vi "checkBeginPassToStrikerPlay.vi"(8 "error in (no error)":errorcluster, 10 "Game":refnum<class "Game.lvclass">, 11 "PassToStriker in":refnum<class "PassToStriker.lvclass">) -> (0 "error out":errorcluster, 2 "result":bool, 3 "PassToStriker out":refnum<class "PassToStriker.lvclass">)   [LabVIEW 2018, in "PassToStrikerPlay.lvclass"]
uses:
  PassToStrikerPlay.lvclass
  temp test/PassToStriker_class/PassToStriker.lvclass
  Game_class/Game.lvclass
  Utilities_class/Utilities.lvclass
  Game_class/Game.lvclass/Game.ctl
  Team_class/Team.lvclass/Team.ctl
  Referee_class/Referee.lvclass/Referee.ctl
  Referee_class/command_interpreted.ctl
  Team_class/OffensivePlay.ctl
  Game_class/Read AllyRef.vi
  Team_class/Read RobotRef.vi
  Game_class/Read Referee.vi
  Referee_class/Read command_interpreted.vi
  Game_class/Read OffensiveTeam.vi
  Team_class/Read OffensivePlay.vi
  Ally_class/Ally.lvclass
  C:/Users/anton/Desktop/roboime/Babulho do Testoni/SSL_AI/Team_class/Team.lvclass
  Referee_class/Referee.lvclass
  Robot_class/Robot.lvclass
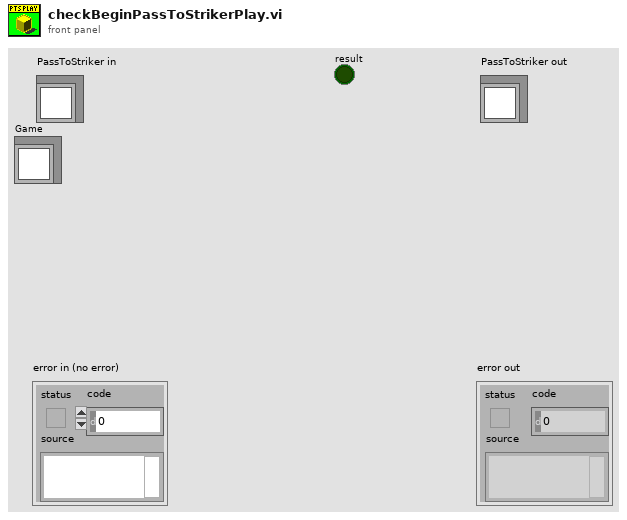
[diagram p1: front panel]
types:
  T1 = typedef "OffensivePlay.ctl" = enum16{"PreparePass", "PassToStriker", "BallOutOfField", "PassTo2ndStriker", "StopOffensive", "Prepare Penalty Enemy", "EnemyPossessionAtEnemyField", "EnemyPossesionAtOurField", "TestPlay", "PreparePenaltyAlly", "KickPenaltyAlly", "PrepareKickoffAlly", "PrepareKickoffEnemy", "IndirectEnemy", "DirectEnemy", "NormalGame", "DirectKick", "Pass", "Halt", "Timeout", "PassPlay", "PenaltyEnemy"}
  T2 = typedef "command_interpreted.ctl" = enum16{"Goal Ally", "Goal Enemy", "Ball Placement Enemy", "Ball Placement Ally", "Normal Half Time", "Extra Time  Break", "Extra Half Time", "None", "Post Game", "PKA Normal Start", "Prepare Kickoff Ally", "PKE Normal Start", "Prepare Kickoff Enemy", "Force Start", "Halt", "Timeout", "Prepare Penalty Ally", "Prepare Penalty Enemy", "PPA NormalStart", "PPE Normal Start", "Indirect Free Ally", "Direct Free Enemy", "Direct Free Ally", "Indirect Free Enemy", "Stop"}
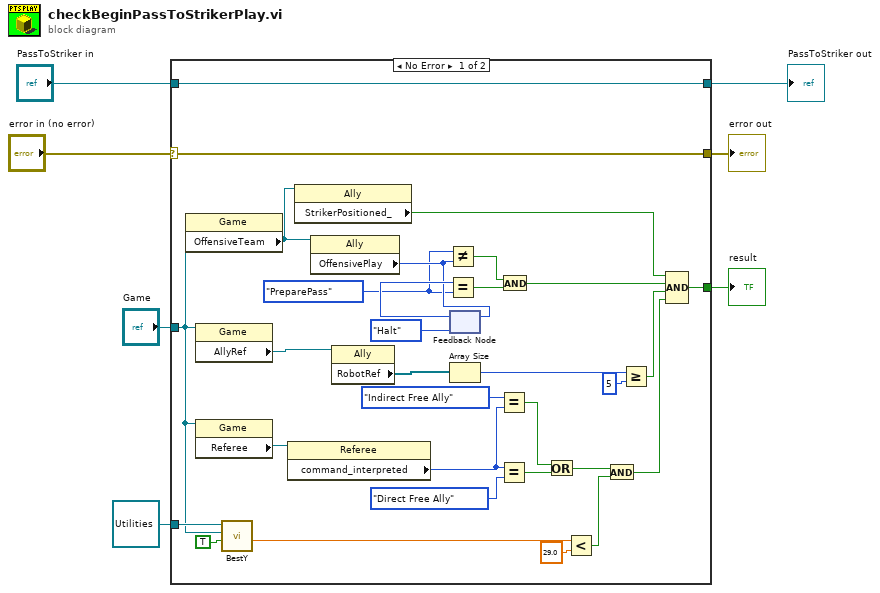
[diagram p0: block diagram]
diagram:
  n1 = case shown="No Error" "error in (no error)" {
    selector: "error in (no error)" -> [w37 w40]
    tunnel: [w37 w40] -> w6
    tunnel: [w38 w39] -> w4
    tunnel: "PassToStriker in" -> [w38 w39]
    tunnel: "Game" -> [w17 _]
    tunnel: refnum<class "Utilities.lvclass"> refnum ("Utilities.lvclass") -> [w25 _]
    tunnel: [w8 _] -> w1
    frame No Error {
      w20 = OffensivePlay."PreparePass" ("OffensivePlay")
      n2 = property class="Game"(reference=w17) -> ("OffensiveTeam"=w24:refnum<class "Ally.lvclass">)  [unwired: 1 in, 2 out]
      n3 = property class="Game"(reference=w17) -> ("AllyRef"=w16:refnum<class "Ally.lvclass">)  [unwired: 1 in, 2 out]
      n4 = property class="Game"(reference=w17) -> ("Referee"=w36:refnum<class "Referee.lvclass">)  [unwired: 1 in, 2 out]
      n5 = call-dynamic "BestY.vi"("Utilities in"=w25, "Game"=w17, "inimigos"=TRUE) -> ("Gap kick"=w28:dbl)  [unwired: 2 in, 4 out]
      n6 = property class="Referee"(reference=w36) -> ("command_interpreted"=w34:T2)  [unwired: 1 in, 2 out]
      n7 = property class="Ally"(reference=w24) -> ("StrikerPositioned_"=w12:bool)  [unwired: 1 in, 2 out]
      n8 = property class="Ally"(reference=w24) -> ("OffensivePlay"=w21:T1)  [unwired: 1 in, 2 out]
      n9 = property class="Ally"(reference=w16) -> ("RobotRef"=w15:refnum<class "Robot.lvclass">[])  [unwired: 1 in, 2 out]
      n10 = Not Equal?(x=w20, y=w21) -> (x != y?=w19:bool)
      n11 = feedback-in #1(w21) -> ()
      n12 = feedback #1(OffensivePlay."Halt" ("OffensivePlay")) -> (w22:T1)
      n13 = Equal?(x=w22, y=w20) -> (x = y?=w18:bool)
      n14 = Array Size(array=w15) -> (size(s)=w14:i32)
      n15 = Equal?(x=command_interpreted."Indirect Free Ally" ("command_interpreted"), y=w34) -> (x = y?=w31:bool)
      n16 = Equal?(x=w34, y=command_interpreted."Direct Free Ally" ("command_interpreted")) -> (x = y?=w32:bool)
      n17 = And(x=w19, y=w18) -> (x .and. y?=w11:bool)
      n18 = Or(x=w31, y=w32) -> (x .or. y?=w26:bool)
      n19 = Less?(x=w28, y=29.0 ("Gap kick")) -> (x < y?=w27:bool)
      n20 = And(x=w26, y=w27) -> (x .and. y?=w9:bool)
      n21 = Greater Or Equal?(x=w14, y=5) -> (x >= y?=w10:bool)
      n22 = Compound Arithmetic op=AND(w12, w11, w10, w9) -> (w8:bool)
    }
    frame Error {
    }
  }
  "error out" <- w6
  "PassToStriker out" <- w4
  "result" <- w1
